vi "imaqdx construct identifier.vi"(11 "Camera Information":T1 {"BusType" format="%x"; "SerialNumberLow" format="%.0x"; "SerialNumberHigh" format="%.0x"}) -> (3 "resulting string":string)   [LabVIEW 2022 SP3, in "Vision.lvlib"]
uses:
  Vision.lvlib
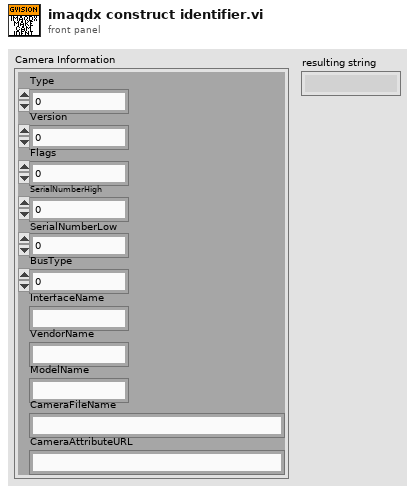
[diagram p1: front panel]
types:
  T1 = cluster{"Type":u32, "Version":u32, "Flags":u32, "SerialNumberHigh":u32, "SerialNumberLow":u32, "BusType":u32, "InterfaceName":string, "VendorName":string, "ModelName":string, "CameraFileName":string, "CameraAttributeURL":string}
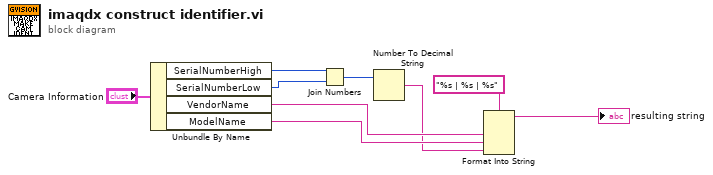
[diagram p0: block diagram]
diagram:
  n1 = Unbundle By Name("Camera Information") -> ("SerialNumberHigh"=w8:u32, "SerialNumberLow"=w7:u32, "VendorName"=w4:string, "ModelName"=w3:string)
  n2 = Join Numbers(hi=w8, lo=w7) -> ((hi.lo)=w6:u64)
  n3 = Number To Decimal String(number=w6) -> (decimal integer string=w2:string)  [unwired: 1 in]
  n4 = Format Into String(format string="%s | %s | %s", w4, w3, w2) -> (resulting string=→"resulting string":string)  [unwired: 2 in, 1 out]
